vi "Print SN.vi"(4 "SN":string="481234501000071600500001") -> ()   [LabVIEW 2009]
uses:
  Global/Global 1.vi
panel:
  out "concatenated string":string
  out "read string":string
  in  "file WEEE":string="WEEE"
  in  "X 5":string="440"
  in  "Y 5":string="4"
  in  "Y 4":string="11"
  in  "X 4":string="490"
  in  "file CE":string="CE"
  in  "Text DOWN":string="0922 SPD 02500"
  in  "X 3":string="260"
  in  "Y 3":string="22"
  in  "Y 2":string="6"
  in  "X 2":string="260"
  in  "Text UP":string="4812345-A-000"
  in  "Y":string="38"
  in  "X":string="260"
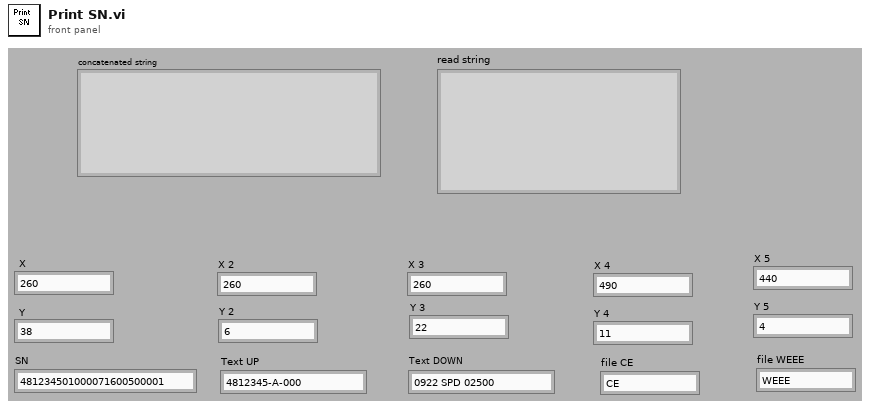
[diagram p1: front panel]
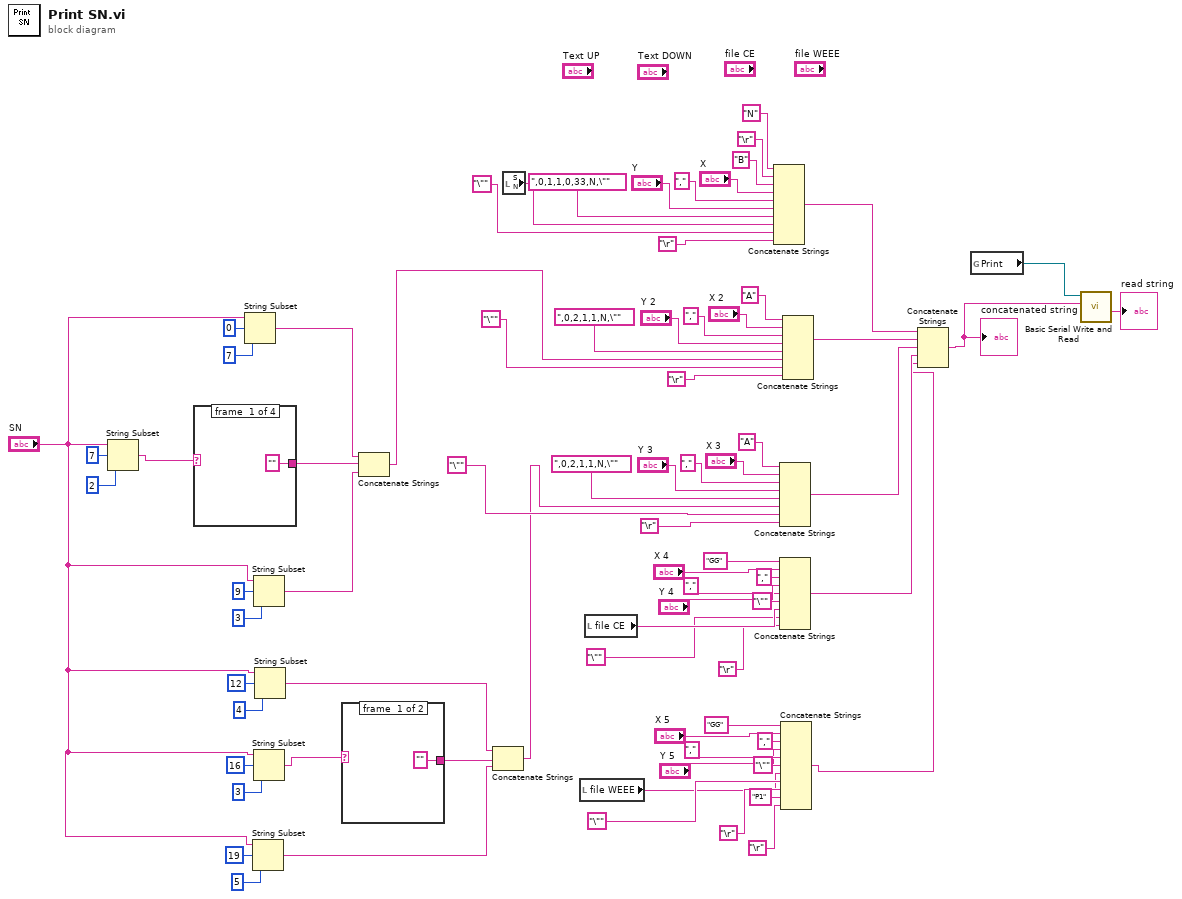
[diagram p0: block diagram]
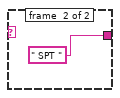
[diagram p2: hidden frame]
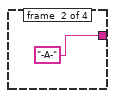
[diagram p3: hidden frame]
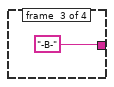
[diagram p4: hidden frame]
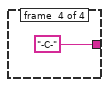
[diagram p5: hidden frame]
diagram:
  n1 = String Subset(string="SN", offset (0)=7, length (rest)=2 ("length (rest)")) -> (substring=w24:string)
  n2 = case shown="\"02\"" w24 {
    tunnel: ["" ("string") "-A-" ("string") "-B-" ("string") "-C-" ("string")] -> w20
    frame #0 {
    }
    frame #1 {
    }
    frame #2 {
    }
    frame #3 {
    }
  }
  n3 = String Subset(string="SN", offset (0)=0, length (rest)=7 ("length (rest)")) -> (substring=w21:string)
  n4 = String Subset(string="SN", offset (0)=19, length (rest)=5 ("length (rest)")) -> (substring=w5:string)
  n5 = String Subset(string="SN", offset (0)=9, length (rest)=3 ("length (rest)")) -> (substring=w17:string)
  n6 = String Subset(string="SN", offset (0)=16, length (rest)=3 ("length (rest)")) -> (substring=w13:string)
  n7 = String Subset(string="SN", offset (0)=12, length (rest)=4 ("length (rest)")) -> (substring=w10:string)
  n8 = case shown="\"005\"" w13 {
    tunnel: ["" ("string") " SPT " ("string")] -> w9
    frame #0 {
    }
    frame #1 {
    }
  }
  n9 = Concatenate Strings(w21, w20, w17) -> (w16:string)
  n10 = Concatenate Strings(w10, w9, w5) -> (w4:string)
  n11 = local read "SN"() -> (w68:string)
  n12 = local read "file WEEE"() -> (w34:string)
  n13 = local read "file CE"() -> (w43:string)
  n14 = Concatenate Strings("N" ("string"), "\r", "B" ("string"), "X", "," ("string"), "Y", ",0,1,1,0,33,N,\"" ("string"), w68, "\"" ("string"), "\r") -> (w58:string)
  n15 = Concatenate Strings("A" ("string"), "X 3", "," ("string"), "Y 3", ",0,2,1,1,N,\"" ("string"), w4, "\"" ("string"), "\r") -> (w50:string)
  n16 = Concatenate Strings("GG" ("string"), "X 4", "," ("string"), "Y 4", "," ("string"), "\"" ("string"), w43, "\"" ("string"), "\r") -> (w39:string)
  n17 = Concatenate Strings("GG" ("string"), "X 5", "," ("string"), "Y 5", "," ("string"), "\"" ("string"), w34, "\"" ("string"), "\r", "P1" ("string"), "\r") -> (w27:string)
  n18 = Concatenate Strings("A" ("string"), "X 2", "," ("string"), "Y 2", ",0,2,1,1,N,\"" ("string"), w16, "\"" ("string"), "\r") -> (w57:string)
  n19 = Concatenate Strings(w58, w57, w50, w39, w27) -> (w3:string)
  "concatenated string" <- w3
  n20 = global read "Global 1.vi" "Print"() -> (w2:refnum<visa-resource-name>)
  n21 = call "Basic Serial Write and Read.vi"("VISA resource name"=w2, "string to write"=w3) -> ("read string"=→"read string":string)  [unwired: 7 in, 1 out]
